vi "Fix Type to GPS Status.vi"(11 "Fix Type":u8) -> (3 "GPS Status":u32)   [LabVIEW 2014]
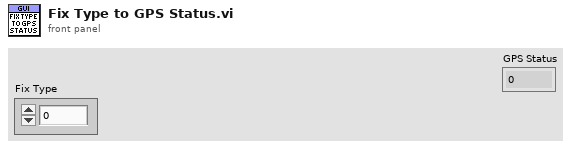
[diagram p1: front panel]
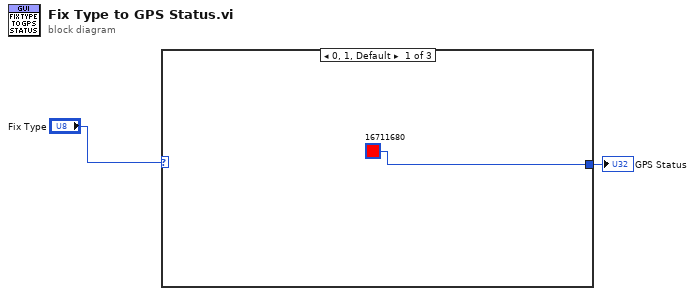
[diagram p0: block diagram]
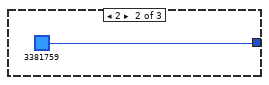
[diagram p2: hidden frame]
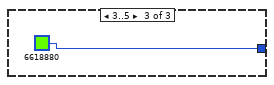
[diagram p3: hidden frame]
diagram:
  n1 = case shown="0, 1, Default" "Fix Type" {
    tunnel: [u32 16711680 u32 3381759 u32 6618880] -> w1
    frame 0, 1, Default {
    }
    frame 2 {
    }
    frame 3..5 {
    }
  }
  "GPS Status" <- w1
